vi "LIN Parameter setzen für Aufzeichnung und Auswertung.vi"(8 "Fehler (Eingang, kein Fehler)":errorcluster, 11 "TestKonfig in":T1 {"TestKonfig Interferent"."Gasflasche MFC3" items=["----"=10000, "IAG NH3 3000"=0, "IAG NH3 200"=1, "IAG NH3 2000"=2, "IAG MG"=3, "IAG O2"=4]; "TestKonfig Interferent"."Gasflasche MFC2" items=["----"=10000, "IAG NH3 3000"=0, "IAG NH3 200"=1, "IAG NH3 2000"=2, "IAG MG"=3, "IAG O2"=4]; "TestKonfig Interferent"."Eingangs Konzentration MFC1" min=0.0; "TestKonfig Interferent"."Ausgangs Konzentration MFC1" min=0.0; "TestKonfig Interferent"."MFC2" items=["MFC 2", "MFC 3", "MFC 4", "MFC 5"]; "TestKonfig Interferent"."MFC3" items=["MFC 2", "MFC 3", "MFC 4", "MFC 5"]; "TestKonfig Interferent"."Ausgangs Konzentration MFC3" min=0.0; "TestKonfig Interferent"."Eingangs Konzentration MFC3" min=0.0; "TestKonfig Interferent"."Ausgangs Konzentration MFC2" min=0.0; "TestKonfig Interferent"."Eingangs Konzentration MFC2" min=0.0; "TestKonfig H2O"."HovaCAL Temperature" format="%.2f"; "TestKonfig H2O"."HovaCAL Flow Input Cluster"."HovaCAL Flow Input Cluster" format="%.2f"; "TestKonfig H2O"."Eingangs Konzentration:" min=0.0; "TestKonfig H2O"."zusätzliche Zeitdauer Erster Punkt" min=30 step=1 format="%#_5g"; "TestKonfig H2O"."Zeitdauer Stufen" format="%#_5g"; "TestKonfig H2O"."Max Fehler" format="%#_5g"; "TestKonfig H2O"."Anzahl Stufen" format="%#_5g"; "TestKonfig H2O"."Modus" items=["Messen", "CG zu Entnahmestelle"]}) -> (0 "Fehler (Ausgang)":errorcluster, 3 "TestKonfig out":T1 {"TestKonfig Interferent"."Gasflasche MFC3" items=["----"=10000, "IAG NH3 3000"=0, "IAG NH3 200"=1, "IAG NH3 2000"=2, "IAG MG"=3, "IAG O2"=4]; "TestKonfig Interferent"."Gasflasche MFC2" items=["----"=10000, "IAG NH3 3000"=0, "IAG NH3 200"=1, "IAG NH3 2000"=2, "IAG MG"=3, "IAG O2"=4]; "TestKonfig Interferent"."Eingangs Konzentration MFC1" min=0.0; "TestKonfig Interferent"."Ausgangs Konzentration MFC1" min=0.0; "TestKonfig Interferent"."MFC2" items=["MFC 2", "MFC 3", "MFC 4", "MFC 5"]; "TestKonfig Interferent"."MFC3" items=["MFC 2", "MFC 3", "MFC 4", "MFC 5"]; "TestKonfig Interferent"."Ausgangs Konzentration MFC3" min=0.0; "TestKonfig Interferent"."Eingangs Konzentration MFC3" min=0.0; "TestKonfig Interferent"."Ausgangs Konzentration MFC2" min=0.0; "TestKonfig Interferent"."Eingangs Konzentration MFC2" min=0.0; "TestKonfig H2O"."HovaCAL Temperature" format="%.2f"; "TestKonfig H2O"."HovaCAL Flow Input Cluster"."HovaCAL Flow Input Cluster" format="%.2f"; "TestKonfig H2O"."Eingangs Konzentration:" min=0.0; "TestKonfig H2O"."zusätzliche Zeitdauer Erster Punkt" min=30 step=1 format="%#_5g"; "TestKonfig H2O"."Zeitdauer Stufen" format="%#_5g"; "TestKonfig H2O"."Max Fehler" format="%#_5g"; "TestKonfig H2O"."Anzahl Stufen" format="%#_5g"; "TestKonfig H2O"."Modus" items=["Messen", "CG zu Entnahmestelle"]})   [LabVIEW 2020, in "EPA 1065.lvlib" / "HovaCAL Interference verificaton.lvlib"]
uses:
  HovaCAL Interference verificaton.lvlib
  TestKonfig.ctl
  TestKonfig H2O.ctl
  Modus.ctl
  Linearisierung V2/SpanEinstellungen/Einheit.ctl
  Linearisierung V2/Gasteiler/Stufen Tabelle.ctl
  Linearisierung V2/Gasteiler/HovaCAL_Interface/Controls/Flow Einstellung.ctl
  Linearisierung V2/Gasteiler/HovaCAL_Interface/Controls/Temp Sollwerte Anzeige.ctl
  TestKonfig Interferents.ctl
  MFCAuswahl.ctl
  Seiten/System Einstellungen V2/Gasflasche Auswahl.ctl
  Linearisierung V2/Aktion Lin Daten aufarbeiten.ctl
  Linearisierung V2/Linearisierung v2.lvlib
  Linearisierung V2/SpanEinstellungen/SpanEinstellungen.lvlib
  Linearisierung V2/Gasteiler/Gasteiler.lvlib
  Linearisierung V2/Gasteiler/HovaCAL_Interface/Controls/Controls.lvlib
  Seiten/System Einstellungen V2/System Einstellungen V2.lvlib
panel:
  # "sec"
  # "%"
  # "sec"
  # "sec"
  # "%"
  # "sec"
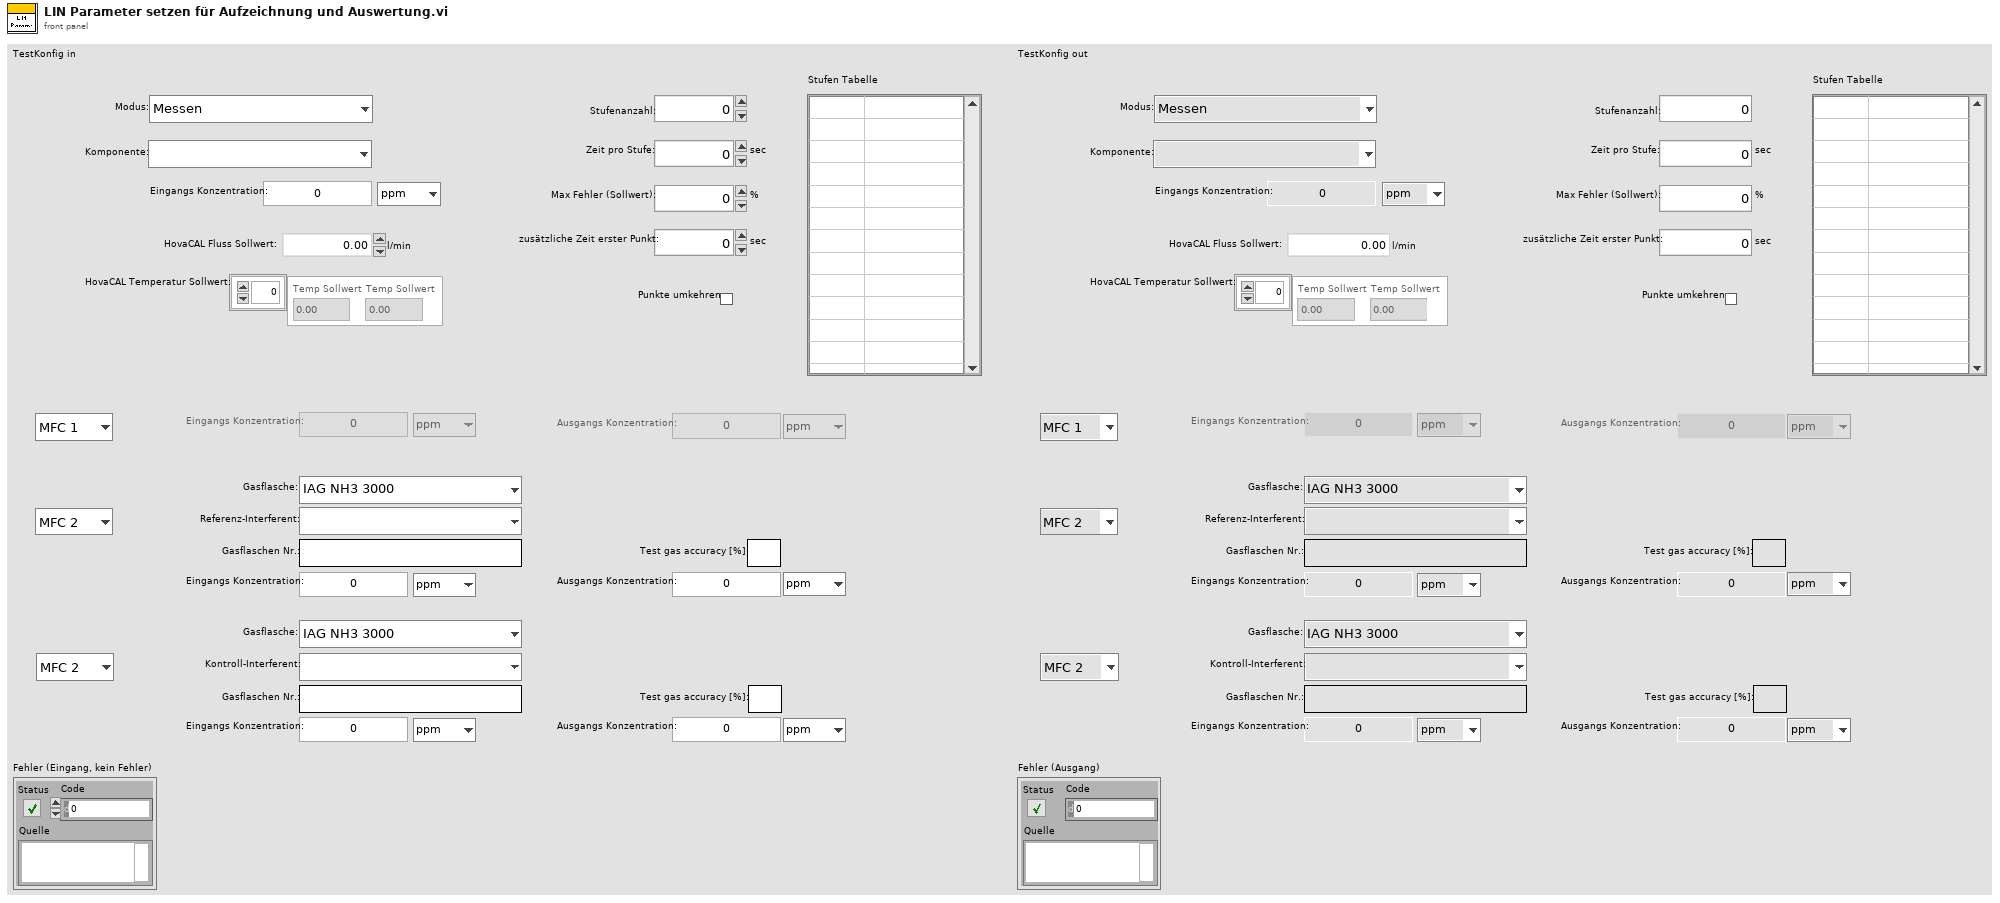
[diagram p1: front panel]
types:
  T1 = typedef "EPA 1065.lvlib/HovaCAL Interference verificaton.lvlib/TestKonfig.ctl" = cluster{"TestKonfig H2O":T2, "TestKonfig Interferent":T8}
  T2 = typedef "EPA 1065.lvlib/HovaCAL Interference verificaton.lvlib/TestKonfig H2O.ctl" = cluster{"Modus":T3, "Komponente:":u16, "Eingangs Konzentration:":dbl, "Einheit":T4, "Anzahl Stufen":sgl, "Zeitdauer Stufen":sgl, "Max Fehler":sgl, "zusätzliche Zeitdauer Erster Punkt":sgl, "Punkte umkehren":bool, "Stufen Tabelle":T5, "HovaCAL Flow Input Cluster":T6, "HovaCAL Temperature":T7}
  T3 = typedef "EPA 1065.lvlib/HovaCAL Interference verificaton.lvlib/Modus.ctl" = u16
  T4 = typedef "Linearisierung v2.lvlib/SpanEinstellungen.lvlib/Einheit.ctl" = enum16{"ppm", "%"}
  T5 = typedef "Linearisierung v2.lvlib/Gasteiler.lvlib/Stufen Tabelle.ctl" = string[][]
  T6 = typedef "Linearisierung v2.lvlib/Gasteiler.lvlib/HovaCAL_Interface.lvlib/Controls.lvlib/Flow Einstellung.ctl" = cluster{"HovaCAL Flow Input Cluster":dbl}
  T7 = typedef "Linearisierung v2.lvlib/Gasteiler.lvlib/HovaCAL_Interface.lvlib/Controls.lvlib/Temp Sollwerte Anzeige.ctl" = dbl[]
  T8 = typedef "EPA 1065.lvlib/HovaCAL Interference verificaton.lvlib/TestKonfig Interferents.ctl" = cluster{"MFC1":enum16{"MFC 1"}, "Eingangs Konzentration MFC1":dbl, "Einheit MFC1 Eingang":T4, "Ausgangs Konzentration MFC1":dbl, "Einheit MFC1 Ausgang":T4, "MFC2":T9, "Referenz-Interferent:":u16, "Gasflaschen Nr MFC2":string, "Accuracy MFC2":string, "Eingangs Konzentration MFC2":dbl, "Einheit MFC2 Eingang":T4, "Ausgangs Konzentration MFC2":dbl, "Einheit MFC2 Ausgang":T4, "MFC3":T9, "Kontroll-Interferent:":u16, "Gasflaschen Nr MFC3":string, "Accuracy MFC3":string, "Eingangs Konzentration MFC3":dbl, "Einheit MFC3 Eingang":T4, "Ausgangs Konzentration MFC3":dbl, "Einheit MFC3 Ausgang":T4, "Gasflasche MFC2":T10, "Gasflasche MFC3":T10}
  T9 = typedef "EPA 1065.lvlib/HovaCAL Interference verificaton.lvlib/MFCAuswahl.ctl" = u16
  T10 = typedef "System Einstellungen V2.lvlib/Gasflasche Auswahl.ctl" = u16
  T11 = typedef "Linearisierung v2.lvlib/Aktion Lin Daten aufarbeiten.ctl" = enum16{"lesen", "Protkolldaten", "speichern", "laden", "EPA auswerten", "Tabelle schreiben", "Lin auswerten", "Tab init", "Stufentabelle", "EPA aktiviert", "Nachbehandlung laden", "Tabelle löschen", "Istwerte löschen", "Zeile löschen", "Zeile einfügen", "LIN aktiviert", "LIN/EPA aktiv laden", "EGAK Tab", "LIN übernehmen", "Tab init ohne Stufen"}
  T12 = cluster{"Komponente:":u16, "Eingangs Konzentration:":dbl}[]
  T13 = typedef "Linearisierung v2.lvlib/Eingabetabelle.ctl" = string[][]
  T14 = typedef "Linearisierung v2.lvlib/Lin-Polynom Daten.ctl" = cluster{"Messgerät":string, "Kalibrator (Gasteiler)":string, "Bearbeiter/in":string, "Komponente":string, "Zeitstempel":timestamp, "F_max gefordert (%)":sgl, "F_max in %":sgl, "F_max in ppm":sgl, "Vorschlag Ordnung":i32, "Polynom OK":bool, "Polynomkoeff.":dbl[], "Prüfgas Konzentration":dbl, "Pfad EPA":string, "Pfad_LIN":string, "Gasnummer:":u8, "Komponentenauswahl":T15, "Verdünnungsgas":T17, "Zeitdauer Stufe":T18, "Anzahl Stufen":T18, "F_max in % EPA":sgl, "F_max in ppm EPA":sgl, "F_max in % LIN":sgl, "F_max in ppm LIN":sgl, "Punkte umkehren":bool, "EPA Optionsfeld":T19, "Autolin Hovacal":T20, "Spanfactors":sgl[], "Kalibrierauswahl":T21, "Conditions:":T22, "Gasflaschen Nr.:":string, "Bottle Accuracy":dbl, "Konfig Gasflasche":T23, "Gasflasche":T10, "HovaCAL Flow AutoLin":T6, "MFC Output":T24, "Gas Ablaufdatum":timestamp, "Lin Modus":T25, "zusätzliche Zeitdauer Erster Punkt":sgl, "Offsets":sgl[]}
  T15 = typedef "Linearisierung v2.lvlib/KomponentenArray.ctl" = cluster{"Komponente:":T16, "Konzentration":dbl}[]
  T16 = typedef "Auswahlfeld.ctl" = u16
  T17 = typedef "Linearisierung v2.lvlib/Gasteiler.lvlib/Prüfgas in.ctl" = u16
  T18 = typedef "Zahlen-Eingabefeld.ctl" = sgl
  T19 = typedef "Linearisierung v2.lvlib/EPA Optionsfeld.ctl" = enum32{"Istwert", "Rohwert", "Linearisierter Wert"}
  T20 = typedef "Linearisierung v2.lvlib/Gasteiler.lvlib/HovaCal.lvlib/AutoLin Hovacal.ctl" = enum32{"Keine Auswahl", "Optionsauswahl 1", "Optionsauswahl 2"}
  T21 = typedef "Linearisierung v2.lvlib/Kalibrieroption.ctl" = u16
  T22 = typedef "Linearisierung v2.lvlib/Linearity verification 1065-307.lvlib/Condition.ctl" = u16
  T23 = typedef "System Einstellungen V2.lvlib/Konfig Gasflasche.ctl" = bool
  T24 = typedef "Linearisierung v2.lvlib/Gasteiler.lvlib/HovaCAL_Interface.lvlib/Controls.lvlib/Pump state.ctl" = cluster{"Run":bool}
  T25 = typedef "CalGas Aufschaltung.lvlib/Lin Modus.ctl" = u16
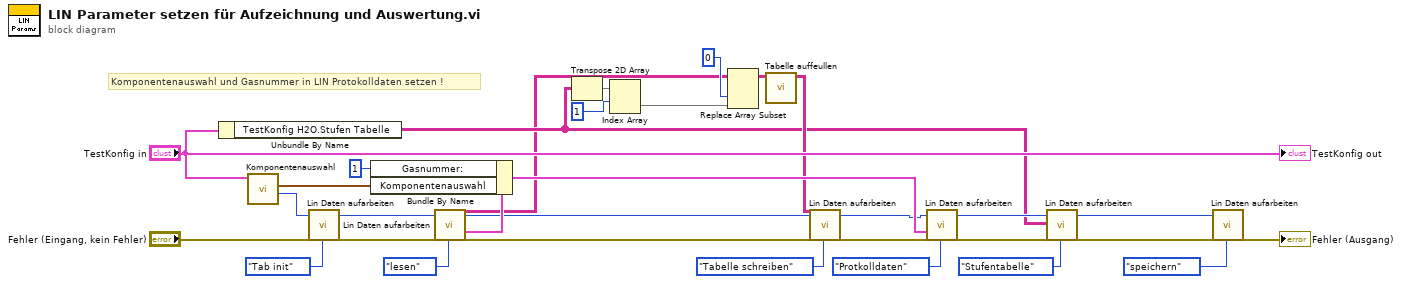
[diagram p0: block diagram]
diagram:
  # "Komponentenauswahl und Gasnummer in LIN Protokolldaten setzen !"
  n1 = Unbundle By Name("TestKonfig in") -> ("TestKonfig H2O.Stufen Tabelle"=w7:T5)
  n2 = call "Komponentenauswahl.vi"("TestKonfig in"="TestKonfig in") -> ("Index absolut"=w19:i32, "Array"=w26:T12)  [unwired: 7 in, 2 out]
  n3 = call "Lin Daten aufarbeiten.vi"("Index (Seite)"=w19, "error in (no error)"="Fehler (Eingang, kein Fehler)", "Aktionen"=Aktion_Lin_Daten_aufarbeiten."Tab init") -> ("Index (Seite) out"=w15:i32, "error out"=w16:errorcluster)  [unwired: 14 in, 9 out]
  n4 = call "Lin Daten aufarbeiten.vi"("Index (Seite)"=w15, "error in (no error)"=w16, "Aktionen"=Aktion_Lin_Daten_aufarbeiten."lesen") -> ("Eingabetabelle"=w5:T13, "Index (Seite) out"=w2:i32, "Lin-Polynom"=w14:T14, "error out"=w4:errorcluster)  [unwired: 14 in, 7 out]
  n5 = Bundle By Name(cluster=w14, "Gasnummer:"=u8 1, "Komponentenauswahl"=w26) -> (w28:T14)
  n6 = Transpose 2D Array(2D array=w7) -> (transposed array=w9:T5)
  n7 = Index Array(array=w9, index (row)=1 ("Index (Zeile)")) -> (element=w6:string[])  [unwired: 1 in]
  n8 = Replace Array Subset(array=w5, new element=w6, index (col)=0 ("Deaktivierter Index (Spalte)")) -> (w12:T13)  [unwired: 1 in]
  n9 = call "Tabelle auffeullen.vi"("Neue Tabelle"=w12) -> ("Tabelle"=w13:string[][])  [unwired: 10 in]
  n10 = call "Lin Daten aufarbeiten.vi"("Eingabetabelle"=w13, "Index (Seite)"=w2, "error in (no error)"=w4, "Aktionen"=Aktion_Lin_Daten_aufarbeiten."Tabelle schreiben") -> ("Index (Seite) out"=w1:i32, "error out"=w3:errorcluster)  [unwired: 13 in, 9 out]
  n11 = call "Lin Daten aufarbeiten.vi"("Index (Seite)"=w1, "Lin-Polynom"=w28, "error in (no error)"=w3, "Aktionen"=Aktion_Lin_Daten_aufarbeiten."Protkolldaten") -> ("Index (Seite) out"=w21:i32, "error out"=w23:errorcluster)  [unwired: 13 in, 9 out]
  n12 = call "Lin Daten aufarbeiten.vi"("Index (Seite)"=w21, "Stufen Tabelle"=w7, "error in (no error)"=w23, "Aktionen"=Aktion_Lin_Daten_aufarbeiten."Stufentabelle") -> ("Index (Seite) out"=w20:i32, "error out"=w22:errorcluster)  [unwired: 13 in, 9 out]
  n13 = call "Lin Daten aufarbeiten.vi"("Index (Seite)"=w20, "error in (no error)"=w22, "Aktionen"=Aktion_Lin_Daten_aufarbeiten."speichern") -> ("error out"=→"Fehler (Ausgang)":errorcluster)  [unwired: 14 in, 10 out]
  "TestKonfig out" <- "TestKonfig in"
